vi "Set Property.vi"(10 "Ctl Ref":refnum<vi>, 11 "Disabled UIP In":refnum<class "DisabledUIP.lvclass">) -> (0 "Error Out":errorcluster, 3 "Disabled UIP Out":refnum<class "DisabledUIP.lvclass">)   [LabVIEW 2015, in "DisabledUIP.lvclass"]
uses:
  DisabledUIP.lvclass
  DisabledUIP.lvclass/DisabledUIP.ctl
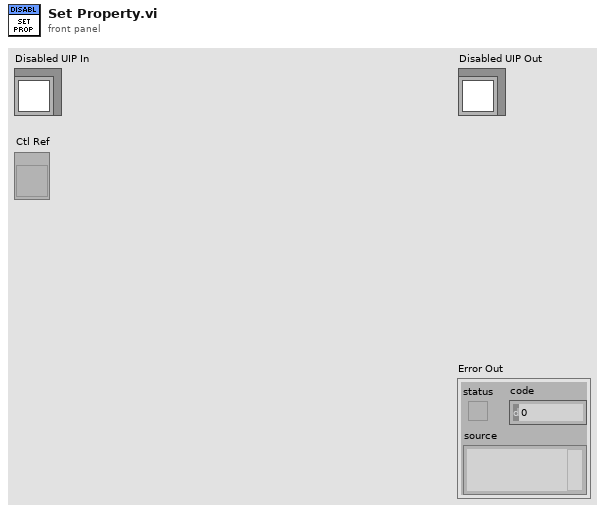
[diagram p1: front panel]
types:
  T1 = enum8{"Enabled", "Disabled", "Disabled and Grayed Out"}
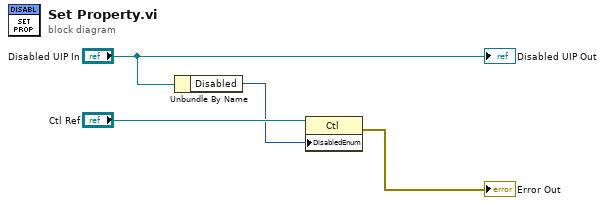
[diagram p0: block diagram]
diagram:
  n1 = Unbundle By Name("Disabled UIP In") -> ("Disabled"=w2:T1)
  n2 = property class="Ctl"(reference="Ctl Ref", "DisabledEnum"=w2) -> (error out=→"Error Out":errorcluster)  [unwired: 1 in, 1 out]
  "Disabled UIP Out" <- "Disabled UIP In"
